vi "Read Sequential Addresses (RolloverDetection).vi"(7 "Target IC (1-8)":u8, 8 "error in (no error)":errorcluster, 9 "Addresses to Read":u16 format="%0.0f", 10 "readConfig":T1 {"upperAddr" format="%04x"; "lowerAddr" format="%04x"; "startAddr" format="%04x"}, 11 "FPGA Interface in":refnum<class "FPGA Interface.lvclass">) -> (0 "error out":errorcluster, 2 "Data":u16[](array[numeric]) format="%04x")   [LabVIEW 2016, in "BCI-1553 API.lvlib" / "FPGA Interface.lvlib" / "FPGA Interface.lvclass"]
uses:
  FPGA Interface.lvclass
  rolloverReadConfig.ctl
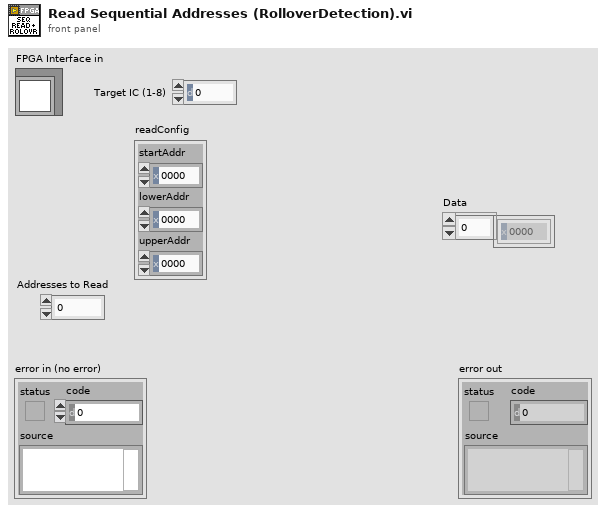
[diagram p1: front panel]
types:
  T1 = typedef "BCI-1553 API.lvlib/FPGA Interface.lvlib/FPGA Interface.lvclass/rolloverReadConfig.ctl" = cluster{"startAddr":u16, "lowerAddr":u16, "upperAddr":u16}
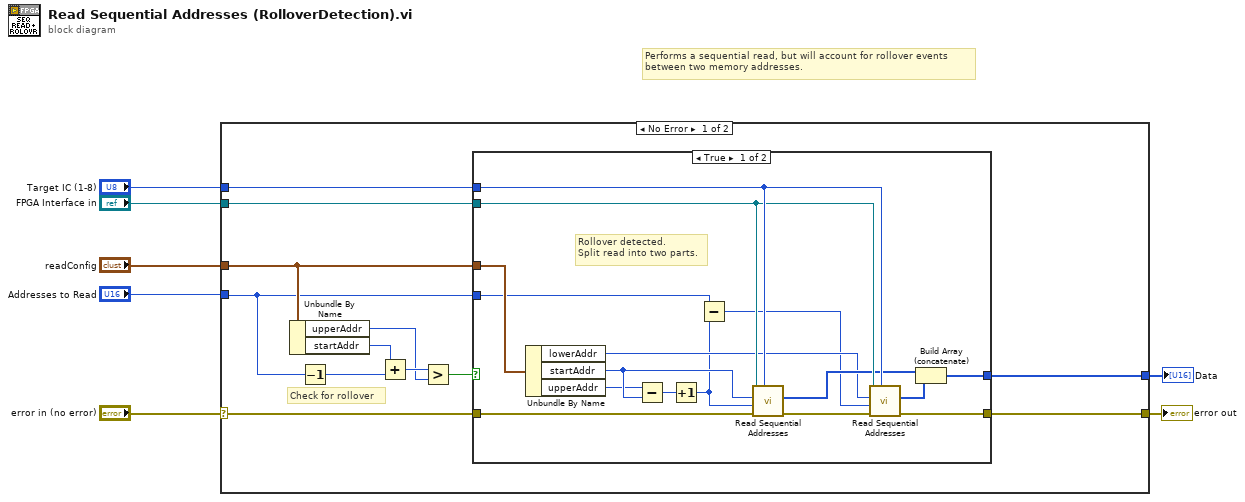
[diagram p0: block diagram]
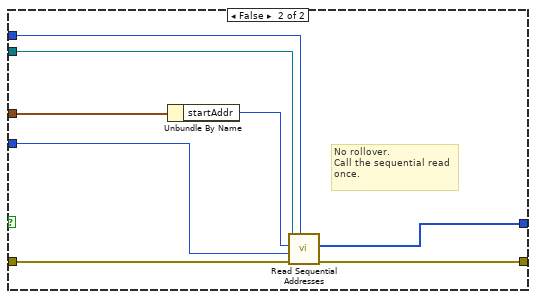
[diagram p2: hidden frame]
diagram:
  # "Performs a sequential read, but will account for rollover events\nbetween two memory addresses."
  n1 = case shown="No Error" "error in (no error)" {
    selector: "error in (no error)" -> [w17 w44]
    tunnel: [w16 w44] -> w6
    tunnel: "FPGA Interface in" -> [w19 _]
    tunnel: "Target IC (1-8)" -> [w18 _]
    tunnel: "readConfig" -> [w10 _]
    tunnel: "Addresses to Read" -> [w9 _]
    tunnel: [w11 _] -> w1
    frame No Error {
      # "Check for rollover"
      n2 = Unbundle By Name(w10) -> ("upperAddr"=w13:u16, "startAddr"=w15:u16)
      n3 = Decrement(x=w9) -> (x-1=w8:u16)
      n4 = Add(x=w15, y=w8) -> (x+y=w14:u16)
      n5 = Greater?(x=w14, y=w13) -> (0:w12:bool)
      n6 = case shown="True" w12 {
        tunnel: w19 -> [w31 w43]
        tunnel: w18 -> [w32 w42]
        tunnel: w17 -> [w35 w41]
        tunnel: [w33 w40] -> w16
        tunnel: [w28 w39] -> w11
        tunnel: w10 -> [w27 w37]
        tunnel: w9 -> [w23 w38]
        frame True {
          # "Rollover detected.\nSplit read into two parts."
          n7 = Unbundle By Name(w27) -> ("lowerAddr"=w24:u16, "startAddr"=w26:u16, "upperAddr"=w25:u16)
          n8 = Subtract(x=w25, y=w26) -> (x-y=w22:u16)
          n9 = Increment(x=w22) -> (x+1=w21:u16)
          n10 = Subtract(x=w23, y=w21) -> (x-y=w20:u16)
          n11 = call-dynamic "Read Sequential Addresses.vi"("Target IC (1-8)"=w32, "error in (no error)"=w35, "Addresses to Read"=w21, "Starting Address"=w26, "FPGA Interface in"=w31) -> ("error out"=w34:errorcluster, "Data"=w30:u16[])  [unwired: 5 in]
          n12 = call-dynamic "Read Sequential Addresses.vi"("Target IC (1-8)"=w32, "error in (no error)"=w34, "Addresses to Read"=w20, "Starting Address"=w24, "FPGA Interface in"=w31) -> ("error out"=w33:errorcluster, "Data"=w29:u16[])  [unwired: 5 in]
          n13 = Build Array (concatenate)(w30, w29) -> (w28:u16[])
        }
        frame False {
          # "No rollover.\nCall the sequential read\nonce."
          n14 = Unbundle By Name(w37) -> ("startAddr"=w36:u16)
          n15 = call-dynamic "Read Sequential Addresses.vi"("Target IC (1-8)"=w42, "error in (no error)"=w41, "Addresses to Read"=w38, "Starting Address"=w36, "FPGA Interface in"=w43) -> ("error out"=w40:errorcluster, "Data"=w39:u16[])  [unwired: 5 in]
        }
      }
    }
    frame Error {
    }
  }
  "error out" <- w6
  "Data" <- w1
